vi "test - Configure Filter.vi"(8 "error in (no error)":errorcluster, 11 "TestCase in":refnum<class "Configure Filter Unit Test.lvclass">) -> (0 "error out":errorcluster, 3 "TestCase out":refnum<class "Configure Filter Unit Test.lvclass">)   [LabVIEW 2017, in "Configure Filter Unit Test.lvclass"]
uses:
  Configure Filter Unit Test.lvclass
  Core/Assert API Components/Filter Configurations/Base Filter.lvclass
  Core/Assert API Components/Filter Configurations/Base Filter.lvclass/Base Filter.ctl
  Configure Filter Unit Test.lvclass/Configure Filter Unit Test.ctl
  <vilib>/addons/_JKI Toolkits/VI Tester/TestCase.llb/TestCase.lvclass
  Core/Main Display/Main Display/Main Display.lvclass
  C:/Program Files (x86)/National Instruments/LabVIEW 2017/vi.lib/addons/_JKI Toolkits/VI Tester/TestCase.llb/TestCase.lvclass
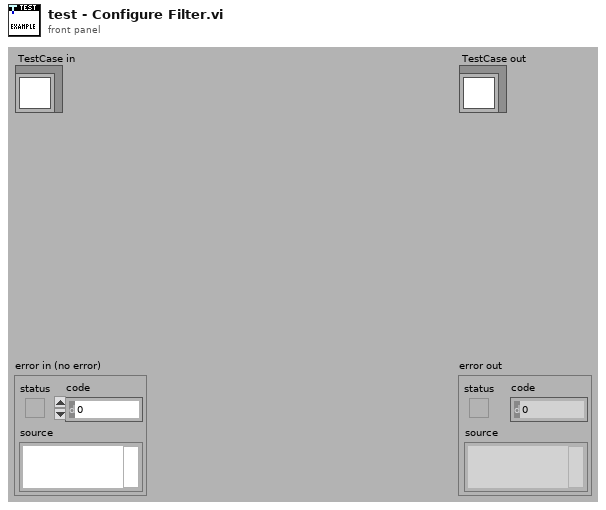
[diagram p1: front panel]
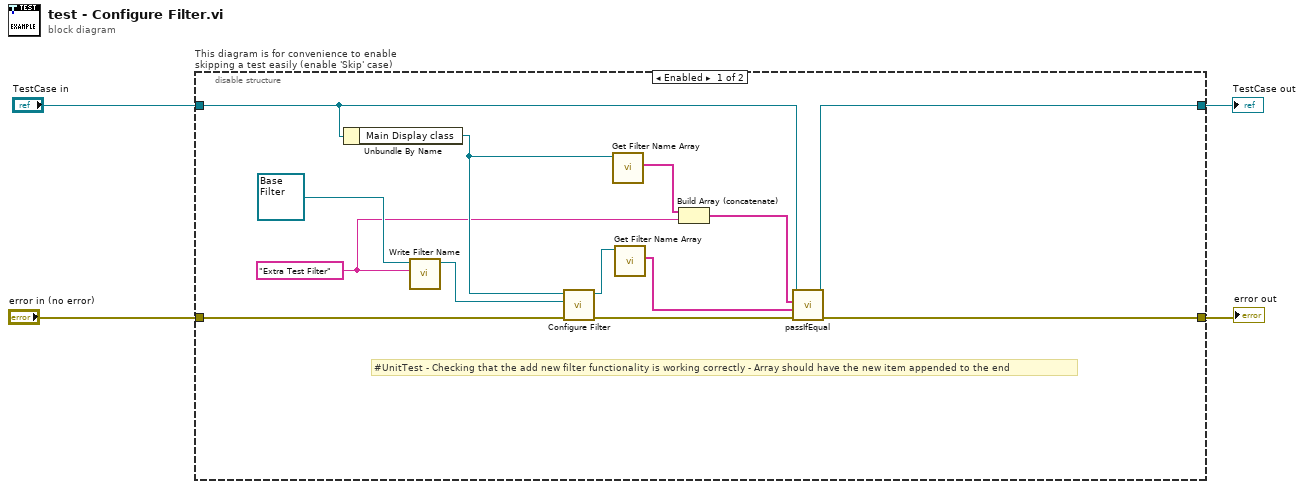
[diagram p0: block diagram]
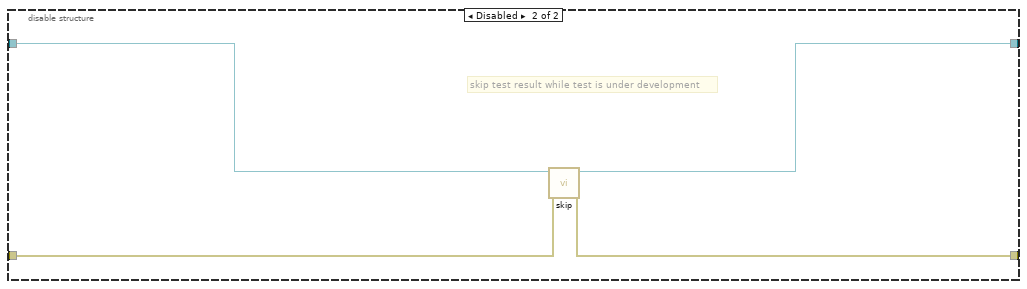
[diagram p2: hidden frame]
diagram:
  n1 = disable-structure "This diagram is for convenience to enable skipping a test easily (enable 'Skip' case)" shown="Enabled" {
    disable-tunnel: "TestCase in" -> [w10 w21]
    disable-tunnel: [w17 w19] -> w1
    disable-tunnel: [w16 w20] -> w3
    disable-tunnel: "error in (no error)" -> [w13 w18]
    frame Enabled {
      w6 = "Extra Test Filter" ("Filter Name")
      # "#UnitTest - Checking that the add new filter functionality is working correctly - Array should have the new item appended to the end"
      n2 = Unbundle By Name(w10) -> ("Main Display class"=w8:refnum<class "Main Display.lvclass">)
      n3 = call "Write Filter Name.vi"("Filter Name"=w6, "Base Filter in"=refnum<class "Base Filter.lvclass"> refnum ("Assert API Components.lvlib:Base Filter.lvclass")) -> ("Base Filter out"=w11:refnum<class "Base Filter.lvclass">)  [unwired: 9 in]
      n4 = call "Configure Filter.vi"("error in (no error)"=w13, "New Filter"=w11, "Main Display in"=w8) -> ("error out"=w12:errorcluster, "Main Display out"=w15:refnum<class "Main Display.lvclass">)  [unwired: 7 in]
      n5 = call "Get Filter Name Array.vi"("Main Display in"=w8) -> ("Filter Name Array"=w7:string[])  [unwired: 10 in]
      n6 = call "Get Filter Name Array.vi"("Main Display in"=w15) -> ("Filter Name Array"=w9:string[])  [unwired: 10 in]
      n7 = Build Array (concatenate)(w7, w6) -> (w5:string[])
      n8 = call-dynamic "passIfEqual.vi"("error in (no error)"=w12, "y"=w9, "x"=w5, "TestCase in"=w10) -> ("error out"=w16:errorcluster, "TestCase out"=w17:refnum<class "Configure Filter Unit Test.lvclass">)  [unwired: 6 in]
    }
    frame Disabled {
      # "skip test result while test is under development"
      n9 = call <vilib>:"skip.vi"("error in (no error)"=w18, "TestCase in"=w21) -> ("error out"=w20:errorcluster, "TestCase out"=w19:refnum<class "Configure Filter Unit Test.lvclass">)  [unwired: 8 in]
    }
  }
  "error out" <- w3
  "TestCase out" <- w1
